vi "Dashboard Main.vi"() -> ()   [LabVIEW 2012]
uses:
  New_Framework_2013/AutoEnum.ctl
  <vilib>/event_ctls.llb/eventvkey.ctl
  <vilib>/Utility/config.llb/Read Key (String).vi
  <vilib>/Utility/config.llb/Read Key (I32).vi
  <vilib>/Utility/config.llb/Write Key (String).vi
  <vilib>/Utility/config.llb/Write Key (I32).vi
  <vilib>/Utility/config.llb/NI_LVConfig.lvlib
panel:
  out "Battery Value":dbl(slide) scale=0.0..14.0 scale format="%#_2e"
  out "Battery":sgl(graph)
  in  "Camera Settings":T1={"Frate Rate"=30, "Compression"=30, "Size"=1} {"Frate Rate" scale=1.0..30.0; "Size" items=["640x480", "320x240", "160x120"]}
  out "Mode":T2(ring)=enum."Auto Disabled"
  out "Camera IP":string
  out "Robot IP":string
  in  "Dashboard Tab":enum32{"Operation", "Test", "Checklist"}(tab)
  out "FrameworkVersion":string
  out "LauncherMotorValue":dbl
  out "Drive Loop Timing (ms)":u32
  out "ClimbState":string
  in  "AutoEnum":T3
  in  "Slider":dbl(slide) scale=0.0..100.0 scale format="%#_3g"
  in  "On/Off":bool caption="Solenoid"
  in  "Test Name":u16(ring) items=["Select the test to run...", "Example Test", "-------------------------------", "List of tests is built in robot code.", "Replace with your own automated tests."]
  in  "Test Tree":string(tree)
  in  "Motor":cluster{"Value":dbl, "Enable":bool} {"Value" scale=-1.0..1.0 scale format="%#_3g"}
  out "Progress":T4 {"Test Progress" scale=0.0..100.0}
  in  "Rev/Fwd":cluster{"Forward":bool, "Reverse":bool}
  in  "Ring":u16(ring) items=["Auto", "Fixed indoor", "Fixed outdoor 1", "Fixed outdoor 2", "Fixed fluorescent 1", "Fixed fluorescent 2", "Hold current"]
  in  "Listbox":i32(listbox)
  in  "Viewer":T5(tab)
  out "Mbps":dbl format="%#.1g"
  in  "Enable":bool
  in  "DB Camera Config":bool
  out "Mbps":bool
  out "fps":dbl format="%#.1g"
  out "Image Error Message":string="Timeout in Camera Communications"
  out "Camera Image":T6(plugin-control)
  out "Buttons 1":cluster{"1":bool, "2":bool, "3":bool}
  out "Kinect 1":cluster{"X":dbl, "Y":dbl, "Z":dbl} {"X" scale=1.0..-1.0; "Y" scale=1.0..-1.0; "Z" scale=1.0..-1.0}
  out "Buttons 2":cluster{"1":bool, "2":bool, "3":bool}
  out "Kinect 2":cluster{"X":dbl, "Y":dbl, "Z":dbl} {"X" scale=1.0..-1.0; "Y" scale=1.0..-1.0; "Z" scale=1.0..-1.0}
  out "Version":string
  out "Skeleton Picture":picture
  out "Players":i8
  out "Tree":string(tree)
  # "Drive & Motors"
  # "Robot IP:"
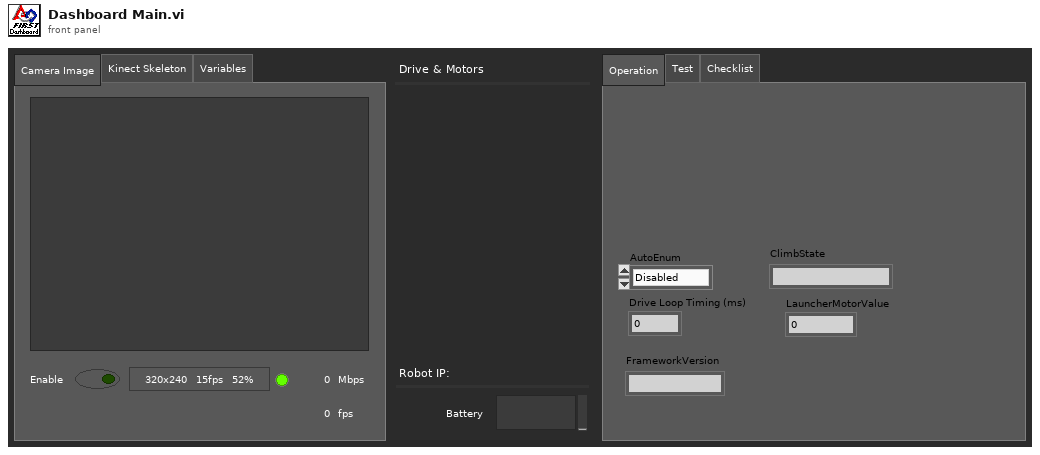
[diagram p1: front panel]
types:
  T1 = cluster{"Frate Rate":i32, "Compression":i32, "Size":u16}
  T2 = enum8{"Tele-Op Disabled", "Tele-Op Enabled", "Auto Disabled", "Auto Enabled", "Test Disabled", "Test Enabled", ""}
  T3 = typedef "AutoEnum.ctl" = enum16{"Disabled", "BackRight", "BackLeft", "CloseRight", "CloseLeft"}
  T4 = cluster{"Test Progress":u8, "Test Progress Text":string}
  T5 = enum32{"Camera Image", "Kinect Skeleton", "Variables"}
  T6 = typedef "IMAQ Image.ctl" = refnum<image>
  T7 = typedef "Image Type" = u32
  T8 = typedef "LVBoundsTypeDef.ctl" = cluster{"Width":u32, "Height":u32}
  T9 = typedef "SkeletonTrackState.ctl" = enum32{"NotTracked", "PositionOnly", "Tracked"}
  T10 = cluster{"TrackingState":u8[], "Position":cluster{"x":sgl, "y":sgl, "z":sgl}, cluster{"x":sgl, "y":sgl, "z":sgl, sgl}[], "TrackState":T9}
  T11 = cluster{cluster{"ScaledToPercentRange":dbl, "ScaledToPercentRange":dbl, "ScaledToPercentRange":dbl}, cluster{bool, bool, bool}}[]
  T12 = cluster{cluster{"ScaledToPercentRange":dbl, "ScaledToPercentRange":dbl, "ScaledToPercentRange":dbl}, cluster{bool, bool, bool}}
  T13 = cluster{"ScaledToPercentRange":dbl, "ScaledToPercentRange":dbl, "ScaledToPercentRange":dbl}
  T14 = typedef "LVRectTypeDef.ctl" = cluster{"Left":i16, "Top":i16, "Right":i16, "Bottom":i16}
  T15 = cluster{"Competition mode":bool, "Robot Link":bool, "Autonomous":bool, "Enabled":bool, "E-Stop":bool, "Simulated":bool, "TestMode":bool, "Docked Window":bool}
  T16 = typedef "NI_LVConfig.lvlib/Config Data RefNum.ctl" = refnum<k1>
  T17 = typedef "eventvkey.ctl" = enum16{"ASCII", "Enter", "Return", "Shift", "Ctrl", "Alt", "Cmd", "Opt", "Caps", "NumLock", "Clear", "Break", "Up", "Down", "Left", "Right", "Insert", "Delete", "Home", "End", "PageUp", "PageDown", "Escape", "Help", "Pause", "ScrollLock", "F1", "F2", "F3", "F4", "F5", "F6", "F7", "F8", "F9", "F10", "F11", "F12", "F13", "F14", "F15", "F16", "F17", "F18", "F19", "F20", "F21", "F22", "F23", "F24", "Play", "VolumeUp", "VolumeDown", "Mute", "Two Byte Char"}
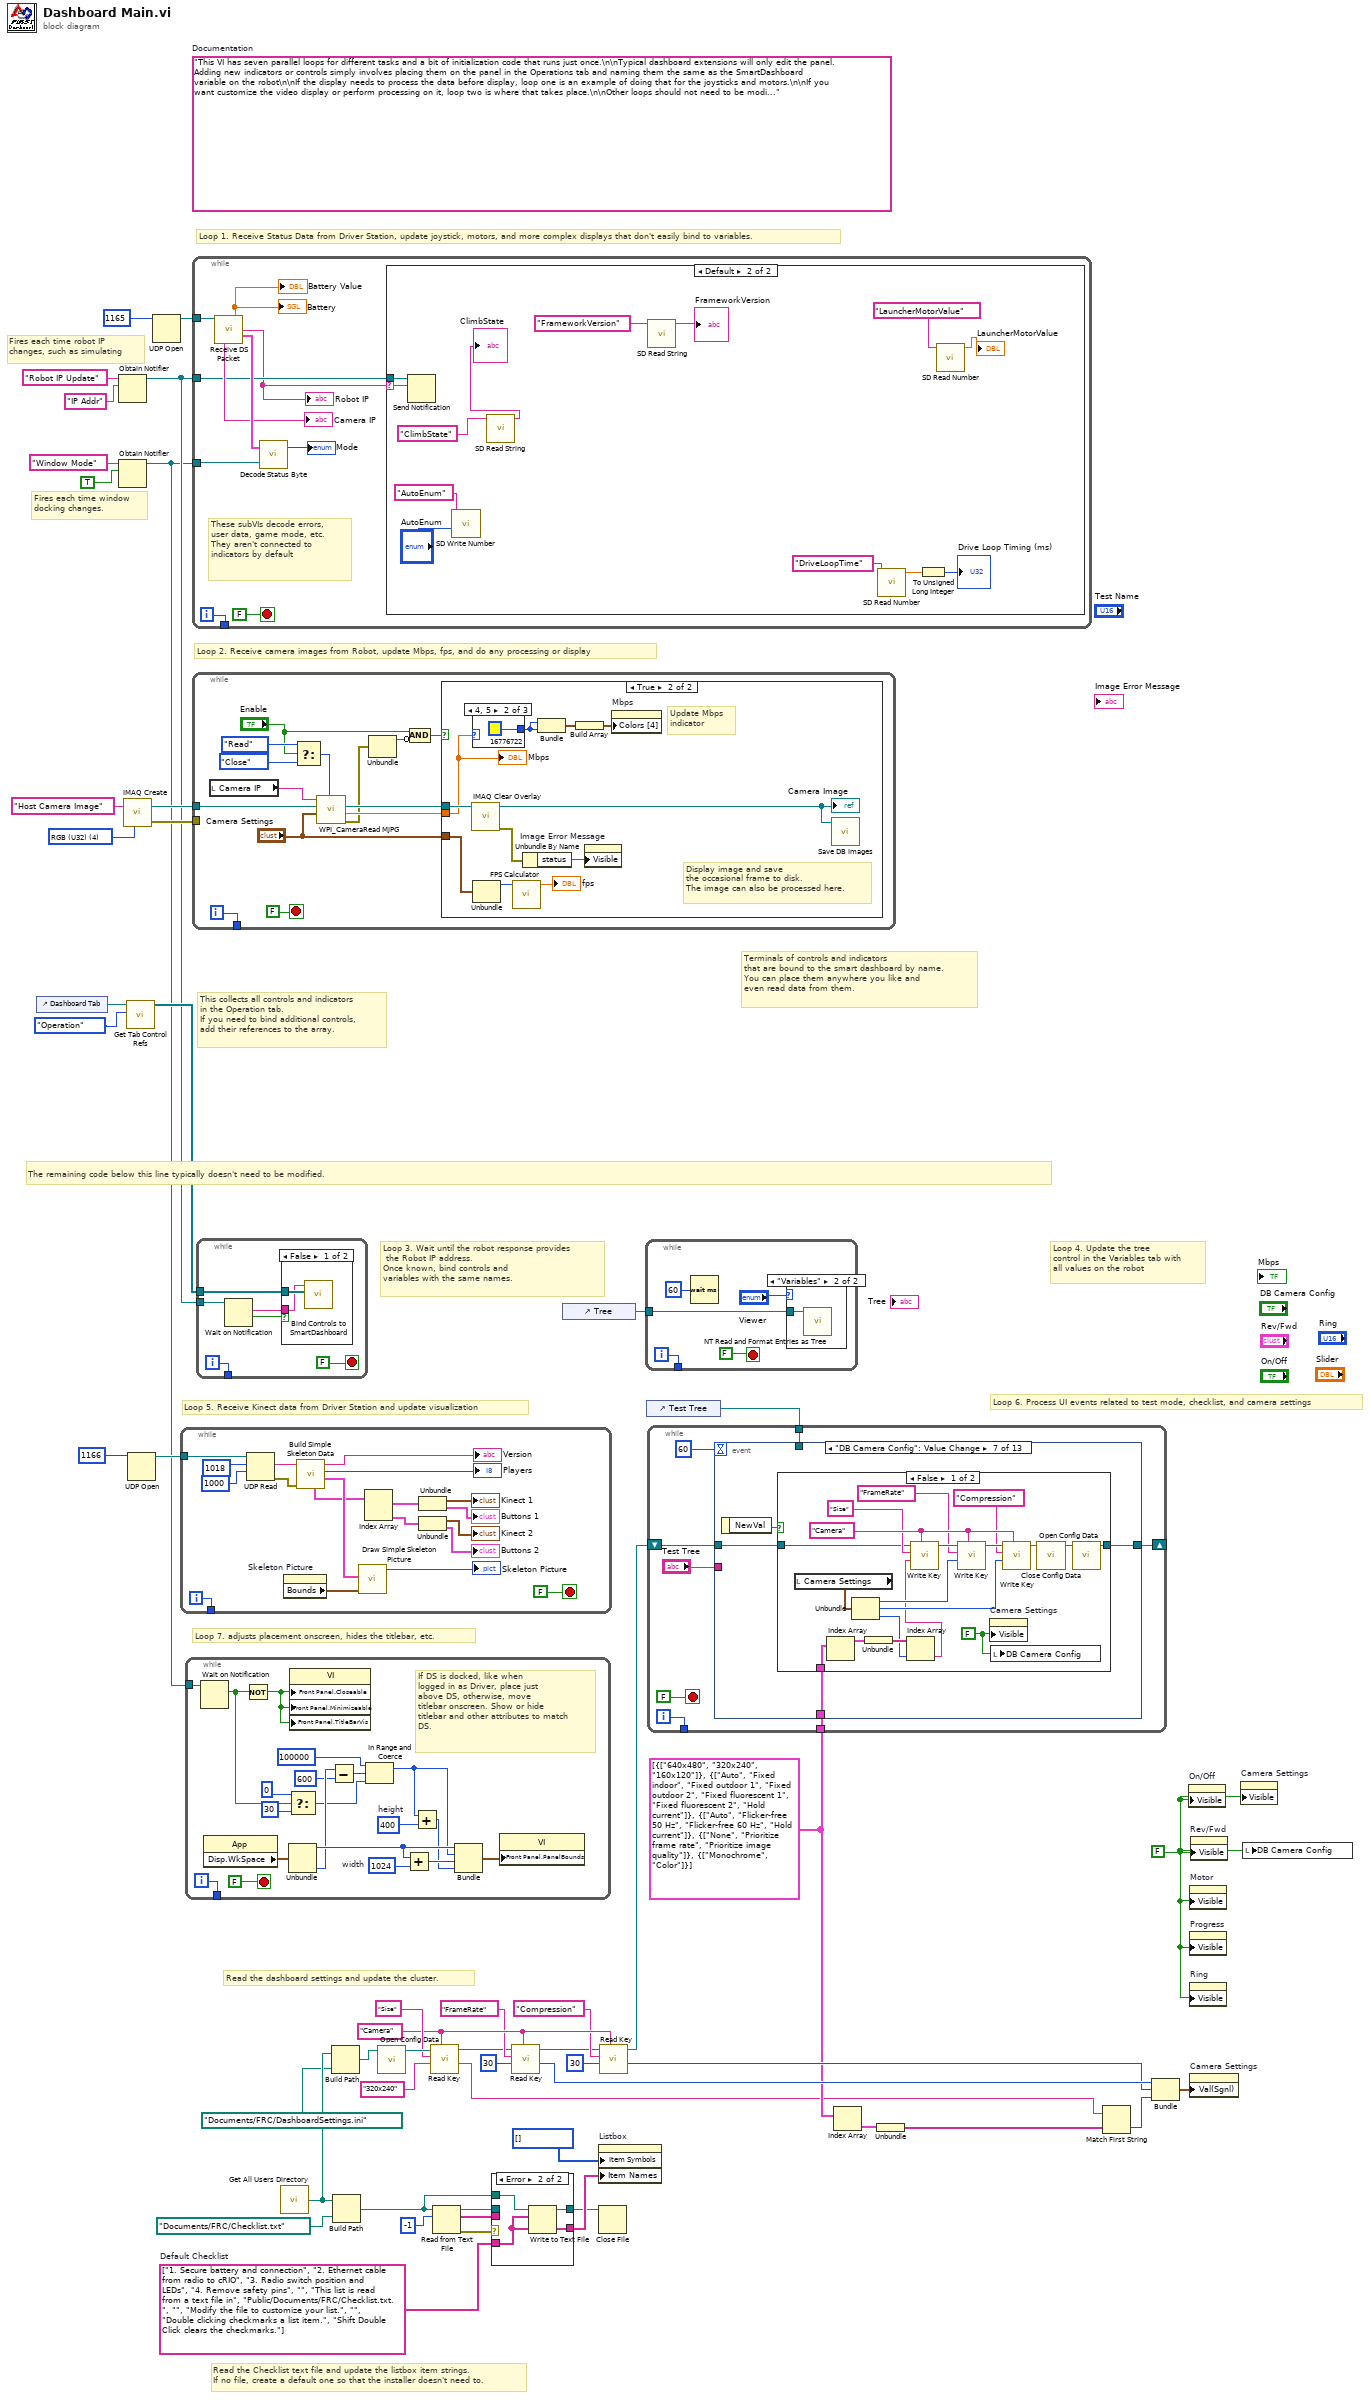
[diagram p0: block diagram]
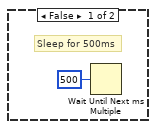
[diagram p3: hidden frame]
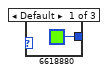
[diagram p4: hidden frame]
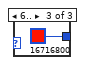
[diagram p5: hidden frame]
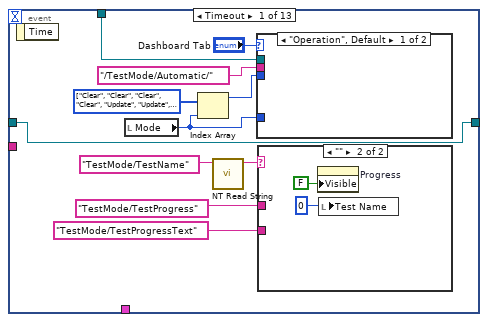
[diagram p7: hidden frame]
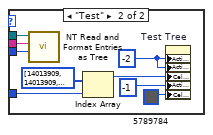
[diagram p8: hidden frame]
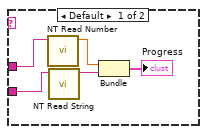
[diagram p9: hidden frame]
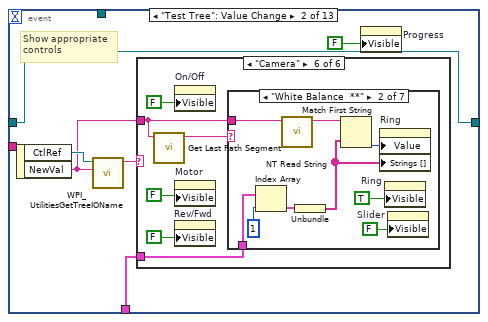
[diagram p10: hidden frame]
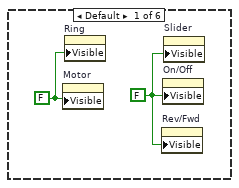
[diagram p11: hidden frame]
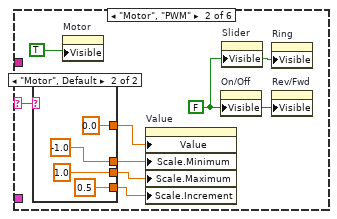
[diagram p12: hidden frame]
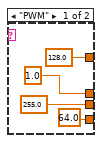
[diagram p13: hidden frame]
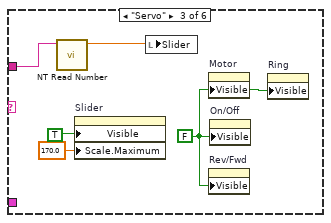
[diagram p14: hidden frame]
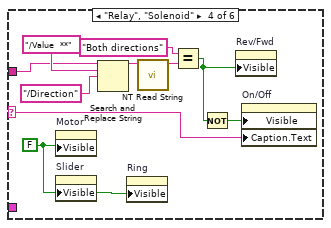
[diagram p15: hidden frame]
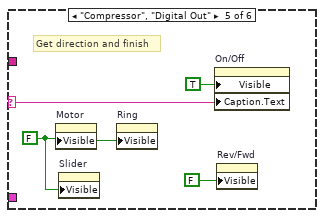
[diagram p16: hidden frame]
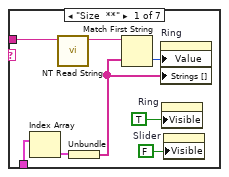
[diagram p17: hidden frame]
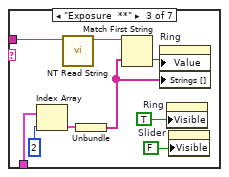
[diagram p18: hidden frame]
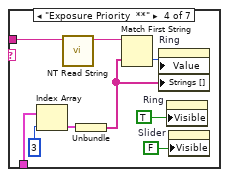
[diagram p19: hidden frame]
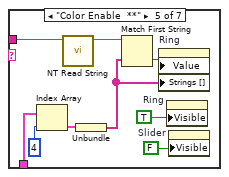
[diagram p20: hidden frame]
diagram:
  w21 = "Camera"
  w13 = cluster{string[]}[] [{["640x480", "320x240", "160x120"]}, {["Auto", "Fixed indoor", "Fixed outdoor 1", "Fixed outdoor 2", "Fixed fluorescent 1", "Fixed fluorescent 2", "Hold current"]}, {["Auto", "Flicker-free 50 Hz", "Flicker-free 60 Hz", "Hold current"]}, {["None", "Prioritize frame rate", "Prioritize image quality"]}, {["Monochrome", "Color"]}]
  w29 = string[] ["1. Secure battery and connection", "2. Ethernet cable from radio to cRIO", "3. Radio switch position and LEDs", "4. Remove safety pins", "", "This list is read from a text file in", "Public/Documents/FRC/Checklist.txt.", "", "Modify the file to customize your list.", "", "Double clicking checkmarks a list item.", "Shift Double Click clears the checkmarks."]  # Default Checklist
  w27 = FALSE ("Visible")
  (unwired) "This VI has seven parallel loops for different tasks and a bit of initialization code that runs just once.\n\nTypical dashboard extensions will only edit the panel. Adding new indicators or controls simply involves placing them on the panel in the Operations tab and naming them the same as the SmartDashboard variable on the robot\n\nIf the display needs to process the data before display, loop one is an example of doing that for the joysticks and motors.\n\nIf you want customize the video display or perform processing on it, loop two is where that takes place.\n\nOther loops should not need to be modified. They are pretty standard, and document the task they perform."  # Documentation
  w50 = T7 4 items=["Grayscale (U8)", "Grayscale (I16)", "Grayscale (SGL)", "Complex (CSG)", "RGB (U32)", "HSL (U32)", "RGB (U64)"] ("Image Type")
  # "Fires each time robot IP\nchanges, such as simulating"
  # "Fires each time window\ndocking changes."
  # "Read the Checklist text file and update the listbox item strings.\nIf no file, create a default one so that the installer doesn't need to."
  # "This collects all controls and indicators\nin the Operation tab.\nIf you need to bind additional controls,\nadd their references to the array."
  # "The remaining code below this line typically doesn't need to be modified."
  # "Loop 6. Process UI events related to test mode, checklist, and camera settings"
  # "Read the dashboard settings and update the cluster."
  # "Terminals of controls and indicators\nthat are bound to the smart dashboard by name.\nYou can place them anywhere you like and\neven read data from them."
  # "Loop 4. Update the tree\ncontrol in the Variables tab with\nall values on the robot"
  # "Loop 3. Wait until the robot response provides\n the Robot IP address.\nOnce known, bind controls and\nvariables with the same names."
  # "Loop 5. Receive Kinect data from Driver Station and update visualization"
  # "Loop 7. adjusts placement onscreen, hides the titlebar, etc."
  # "Loop 1. Receive Status Data from Driver Station, update joystick, motors, and more complex displays that don't easily bind to variables."
  # "Loop 2. Receive camera images from Robot, update Mbps, fps, and do any processing or display"
  n1 = control-ref of="Dashboard Tab"() -> (w43:refnum<vi>)
  n2 = Obtain Notifier(name (unnamed)="Robot IP Update", notification data type="IP Addr" ("name (unnamed)")) -> (notifier out=w40:refnum<notifier>)  [unwired: 2 in, 2 out]
  n3 = Obtain Notifier(name (unnamed)="Window Mode", notification data type=TRUE) -> (notifier out=w33:refnum<notifier>)  [unwired: 2 in, 2 out]
  n4 = call "IMAQ Create"("Image Name"="Host Camera Image", "Image Type"=w50) -> ("New Image"=w48:T6, "error out"=w47:errorcluster)  [unwired: 2 in, 1 out]
  n5 = call <vilib>:"Get Tab Control Refs.vi"("Page Index"=enum32{"Operation", "Test"}."Operation" ("Dashboard Tab"), "TabControl in"=w43) -> ("ControlsOnPage"=w44:refnum<vi>[])  [unwired: 9 in]
  n6 = UDP Open(11:u16 1166 ("port")) -> (port=w45:refnum<k16>)  [unwired: 2 in, 4 out]
  n7 = UDP Open(11:u16 1165 ("port")) -> (port=w51:refnum<k16>)  [unwired: 2 in, 4 out]
  n8 = while {
    tunnel: w45 -> [w69]
    tunnel: [w54] -> _
    i -> [w54]
    stop <- FALSE stop-if-true
    n9 = UDP Read(connection ID=w69, max size (548)=1018 ("bytes to read"), timeout ms (25000)=1000) -> (data out=w63:string, error out=w53:errorcluster)  [unwired: 1 in, 3 out]
    n10 = property on="Skeleton Picture" class="Pict"() -> ("Bounds"=w65:T8)  [unwired: 2 in, 2 out]
    n11 = call "Build Simple Skeleton Data.vi"("error in (no error)"=w53, "data in"=w63) -> ("Skeleton Data"=w64:T10, "NumPlayers"=→"Players":i8, "Version String"=→"Version":string, "Simple Joystick Info"=w61:T11)  [unwired: 5 in, 1 out]
    n12 = call "Draw Simple Skeleton Picture.vi"("Bounds"=w65, "Simple Skeleton"=w64) -> ("new picture out"=→"Skeleton Picture":picture)  [unwired: 9 in]
    n13 = Index Array(array=w61) -> (element #1=w60:T12, element #2=w59:T12)  [unwired: 2 in]
    n14 = Unbundle(w60) -> (→"Kinect 1":T13, →"Buttons 1":cluster{bool, bool, bool})
    n15 = Unbundle(w59) -> (→"Kinect 2":T13, →"Buttons 2":cluster{bool, bool, bool})
  }
  n16 = while {
    tunnel: w33 -> [w90]
    tunnel: [w88] -> _
    i -> [w88]
    stop <- FALSE stop-if-true
    w80 = 1024  # width
    w83 = 400  # height
    # "If DS is docked, like when\nlogged in as Driver, place just\nabove DS, otherwise, move\ntitlebar onscreen. Show or hide\ntitlebar and other attributes to match\nDS."
    n17 = Wait on Notification(notifier=w90) -> (notification=w75:bool)  [unwired: 3 in, 3 out]
    n18 = property class="App"() -> ("Disp.WkSpace"=w86:T14)  [unwired: 2 in, 2 out]
    n19 = Not(x=w75) -> (.not. x?=w89:bool)
    n20 = Unbundle(w86) -> ("Left"=w84:i16, "Bottom"=w81:i16)  [unwired: 2 out]
    n21 = Select(t=0, s=w75, f=30) -> (s? t:f=w74:i32)
    n22 = property class="VI"("Front Panel.Closeable"=w89, "Front Panel.Minimizeable"=w89, "Front Panel.TitleBarVis"=w89) -> ()  [unwired: 2 in, 2 out]
    n23 = Subtract(x=w81, y=600) -> (x-y=w78:i32)
    n24 = In Range and Coerce(upper limit=100000, x=w78, lower limit=w74) -> (coerced(x)=w72:i32)  [unwired: 1 out]
    n25 = Add(x=w84, y=w80) -> (x+y=w85:i32)
    n26 = Add(x=w72, y=w83) -> (x+y=w82:i32)
    n27 = Bundle("Left"=w84, w72, w85, w82) -> (w87:cluster{"Left":i16, i32, i32, i32})  [unwired: 1 out]
    n28 = property class="VI"("Front Panel.PanelBounds"=w87) -> ()  [unwired: 2 in, 2 out]
  }
  n29 = while {
    tunnel: w48 -> [w101]
    tunnel: w47 -> [_]
    tunnel: [w104] -> _
    i -> [w104]
    stop <- FALSE stop-if-true
    n30 = local read "Camera IP"() -> (w103:string)
    n31 = Select(t=enum16{"Read", "Reopen", "Close"}."Read" ("Operation"), s="Enable", f=enum16{"Read", "Reopen", "Close"}."Close" ("Operation")) -> (s? t:f=w96:enum16{"Read", "Reopen", "Close"})
    n32 = call <vilib>:"WPI_CameraRead MJPG.vi"("Operation"=w96, "Camera Settings"="Camera Settings", "Image"=w101, "address"=w103) -> ("error out"=w95:errorcluster, "Bandwidth (kbps)"=w99:dbl, "Image Out"=w100:T6)  [unwired: 5 in]
    n33 = Unbundle(w95) -> ("status"=w93:bool)  [unwired: 2 out]
    n34 = Compound Arithmetic op=AND("Enable", invert w93) -> (w92:bool)
    n35 = case shown="True" w92 {
      tunnel: "Camera Settings" -> [_ w108]
      tunnel: w100 -> [_ w111]
      tunnel: w99 -> [_ w110]
      frame False {
        # "Sleep for 500ms"
        n36 = Wait Until Next ms Multiple(millisecond multiple=u32 500) -> ()  [unwired: 1 out]
      }
      frame True {
        # "Display image and save\nthe occasional frame to disk.\nThe image can also be processed here."
        # "Update Mbps\nindicator"
        n37 = call "IMAQ Clear Overlay"("Image"=w111) -> ("error out"=w116:errorcluster, "Image Out"=w115:T6)  [unwired: 2 in, 7 out]
        "Camera Image" <- w115
        n38 = case shown="4, 5" w110 {
          tunnel: [u32 6618880 ("Color Box") u32 16776722 ("Color Box") u32 16716800 ("Color Box")] -> w112
          frame Default {
          }
          frame 4, 5 {
          }
          frame 6.. {
          }
        }
        n39 = Unbundle(w108) -> ("Frate Rate"=w107:i32)  [unwired: 2 out]
        n40 = call "FPS Calculator.vi"("Average Count"=w107) -> ("fps"=→"fps":dbl)  [unwired: 10 in]
        n41 = Unbundle By Name(w116) -> ("status"=w117:bool)
        n42 = Bundle("Color Box"=w112, "Color Box"=w112) -> (w114:cluster{"Color Box":u32, "Color Box":u32})  [unwired: 1 out]
        n43 = Build Array(w114) -> (w113:cluster{"Color Box":u32, "Color Box":u32}[])
        n44 = property on="Image Error Message" class="Str"("Visible"=w117) -> ()  [unwired: 2 in, 2 out]
        n45 = property on="Mbps" class="Bool (strict)"("Colors [4]"=w113) -> ()  [unwired: 2 in, 2 out]
        n46 = call "Save DB Images.vi"("Image"=w115) -> ()  [unwired: 2 in, 1 out]
        "Mbps" <- w110
      }
    }
  }
  n47 = while {
    tunnel: w51 -> [w128]
    tunnel: w40 -> [w122]
    tunnel: w33 -> [w126]
    tunnel: [w123] -> _
    i -> [w123]
    stop <- FALSE stop-if-true
    # "These subVIs decode errors, user data, game mode, etc.\nThey aren't connected to indicators by default"
    n48 = call "Receive DS Packet.vi"("Recv Socket"=w128) -> ("Battery"=→"Battery" →"Battery Value":sgl, "Robot IP Address"=w121:string, "Status"=w129:T15, "Camera IP Address"=→"Camera IP":string)  [unwired: 1 in, 10 out]
    "Robot IP" <- w121
    n49 = call "Decode Status Byte.vi"("Window Mode Notifier"=w126, "Status"=w129) -> ("Mode"=→"Mode":T2)  [unwired: 1 out]
    n50 = case shown="Default" w121 {
      selector: w121 -> [_ w142]
      tunnel: w122 -> [_ w143]
      frame "0.0.0.0" {
        # "Robot not responding, don't poll the variables"
      }
      frame Default {
        n51 = Send Notification(notification=w142, notifier=w143) -> ()  [unwired: 1 in, 2 out]
        n52 = call <vilib>:"SD Write Number.vi"("Numeric"="AutoEnum", "Name"="AutoEnum") -> ()  [unwired: 8 in, 2 out]
        n53 = call <vilib>:"SD Read String.vi"("Name"="ClimbState") -> ("String"=→"ClimbState":string)  [unwired: 8 in, 2 out]
        n54 = call <vilib>:"SD Read String.vi"("Name"="FrameworkVersion") -> ("String"=→"FrameworkVersion":string)  [unwired: 8 in, 2 out]
        n55 = call <vilib>:"SD Read Number.vi"("Name"="DriveLoopTime") -> ("Numeric"=w137:dbl)  [unwired: 8 in, 2 out]
        n56 = To Unsigned Long Integer(number=w137) -> (unsigned 32bit integer=→"Drive Loop Timing (ms)":u32)
        n57 = call <vilib>:"SD Read Number.vi"("Name"="LauncherMotorValue") -> ("Numeric"=→"LauncherMotorValue":dbl)  [unwired: 8 in, 2 out]
      }
    }
  }
  n58 = while {
    tunnel: w44 -> [w149]
    tunnel: w40 -> [w146]
    tunnel: [w144] -> _
    i -> [w144]
    stop <- FALSE stop-if-true
    n59 = Wait on Notification(notifier=w146) -> (notification=w145:string, timed out?=w147:bool)  [unwired: 3 in, 2 out]
    n60 = case shown="False" w147 {
      tunnel: w149 -> [w151 _]
      tunnel: w145 -> [w150 _]
      frame False {
        n61 = call <vilib>:"Bind Controls to SmartDashboard.vi"("Bound Control Refs"=w151, "Server IP Address"=w150) -> ()  [unwired: 10 in]
      }
      frame True {
      }
    }
  }
  n62 = call "Get All Users Directory.vi"() -> ("All User Path"=w26:path)
  n63 = Build Path(base path=w26, name or relative path=path "Documents/FRC/DashboardSettings.ini") -> (appended path=w25:path)
  n64 = Build Path(base path=w26, name or relative path=path "Documents/FRC/Checklist.txt") -> (appended path=w30:path)
  n65 = call <vilib>:"Open Config Data.vi"("configuration file path"=w25) -> ("refnum"=w24:T16)  [unwired: 8 in, 2 out]
  n66 = call-poly <vilib>:"Read Key.vi"("section"=w21, "default value"="320x240", "key"="Size", "refnum"=w24) -> ("value"=w11:string, "refnum out"=w6:T16)  [unwired: 2 in, 4 out]
  n67 = Read from Text File(file (use dialog)=w30, count=-1 ("timeout ms (25000)")) -> (refnum out=w8:refnum<file>, text=w31:string[], error out=w32:errorcluster)  [unwired: 2 in, 1 out]
  n68 = case shown="Error" w32 {
    tunnel: w31 -> [w153 _]
    tunnel: [w153 w155] -> w28
    tunnel: w29 -> [_ w155]
    tunnel: w30 -> [_ w156]
    tunnel: [w152 w154] -> w7
    tunnel: w8 -> [w152 _]
    frame No Error {
    }
    frame Error {
      n69 = Write to Text File(file (use dialog)=w156, text=w155) -> (refnum out=w154:refnum<file>)  [unwired: 2 in, 2 out]
    }
  }
  n70 = call-poly <vilib>:"Read Key.vi"("section"=w21, "default value"=30, "key"="FrameRate", "refnum"=w6) -> ("value"=w16:i32, "refnum out"=w5:T16)  [unwired: 1 in, 5 out]
  n71 = control-ref of="Tree"() -> (w2:refnum<vi>)
  n72 = property on="Listbox" class="LstBox (strict)"("Item Symbols"=i32[] [], "Item Names"=w28) -> ()  [unwired: 2 in, 2 out]
  n73 = Close File(refnum=w7) -> ()  [unwired: 1 in, 2 out]
  n74 = call-poly <vilib>:"Read Key.vi"("section"=w21, "default value"=30, "key"="Compression", "refnum"=w5) -> ("value"=w15:i32, "refnum out"=w3:T16)  [unwired: 1 in, 5 out]
  n75 = while {
    tunnel: [w158] -> _
    tunnel: w2 -> [w157]
    i -> [w158]
    stop <- FALSE stop-if-true
    n76 = Wait (ms)(milliseconds to wait=u32 60) -> ()  [unwired: 1 out]
    n77 = case shown="\"Variables\"" "Viewer" {
      tunnel: w157 -> [_ w162]
      frame Default {
      }
      frame "Variables" {
        n78 = call <vilib>:"NT Read and Format Entries as Tree.vi"("Tree Refnum"=w162) -> ()  [unwired: 9 in, 2 out]
      }
    }
  }
  n79 = control-ref of="Test Tree"() -> (w1:refnum<vi>)
  n80 = while {
    tunnel: w13 -> [w167]
    shift-right: [w166] -> _
    shift-left: w3 -> [w165]
    tunnel: [w164] -> _
    tunnel: w1 -> [w163]
    i -> [w164]
    stop <- FALSE stop-if-true
    n81 = event shown="[6] \"DB Camera Config\": Value Change" {
      selector: _ -> [_ _ _ _ _ _ _ _ _ _ _ _ _]
      dyn-events: _ -> [_ _ _ _ _ _ _ _ _ _ _ _ _]
      timeout: u32 60 ("milliseconds to wait") -> [_ _ _ _ _ _ _ _ _ _ _ _ _]
      tunnel: w163 -> [w177 _ _ _ _ _ _ _ _ _ _ _ _]
      tunnel: "Test Tree" -> [_ _ _ _ _ _ _ _ w371 w379 w381 w385 w393]
      tunnel: w167 -> [_ w199 _ _ _ _ w335 w365 _ _ _ _ _]
      tunnel: [w171 w198 _ w301 w309 w321 w334 w358 w370 w377 w380 w384 w392] -> w166
      tunnel: w165 -> [w171 w198 _ w301 w309 w321 w333 w358 w370 w377 w380 w384 w392]
      event Timeout {
        w176 = enum16{"Update", "Clear"}[] [enum."Clear", enum."Clear", enum."Clear", enum."Clear", enum."Update", enum."Update", enum."Clear"] items=["Update", "Clear"]
        n82 = event-data() -> ()  [unwired: 1 in, 1 out]
        n83 = local read "Mode"() -> (w174:T2)
        n84 = Index Array(array=w176, index=w174) -> (element=w175:enum16{"Update", "Clear"})
        n85 = call <vilib>:"NT Read String.vi"("Name"="TestMode/TestName") -> ("String"=w180:string)  [unwired: 9 in, 1 out]
        n86 = case shown="\"Operation\", Default" "Dashboard Tab" {
          tunnel: w177 -> [_ w190]
          tunnel: "/TestMode/Automatic/" ("Name Pattern") -> [_ w189]
          tunnel: w175 -> [_ w188]
          tunnel: w174 -> [_ w186]
          frame "Operation", Default {
          }
          frame "Test" {
            w185 = -2 ("Active Item:Row Number")
            n87 = call <vilib>:"NT Read and Format Entries as Tree.vi"("Operation"=w188, "Name Pattern"=w189, "Tree Refnum"=w190) -> ()  [unwired: 7 in, 2 out]
            n88 = Index Array(array=u32[] [14013909, 14013909, 14013909, 14013909, 14013909, 16777215, 14013909], index=w186) -> (element=w184:u32)
            n89 = property on="Test Tree" class="Tree (strict)"("Active Item Row Number"=w185, "ActiveColNum"=w185, "CellBG"=w184, "Active Item Row Number"=-1 ("Active Item:Row Number"), "CellBG"=u32 5789784 ("Color Box")) -> ()  [unwired: 2 in, 2 out]
          }
        }
        n90 = case shown="\"\"" w180 {
          tunnel: "TestMode/TestProgress" ("Name") -> [w192 _]
          tunnel: "TestMode/TestProgressText" ("Name") -> [w191 _]
          frame Default {
            n91 = call <vilib>:"NT Read Number.vi"("Name"=w192) -> ("Numeric"=w193:dbl)  [unwired: 9 in, 1 out]
            n92 = call <vilib>:"NT Read String.vi"("Name"=w191) -> ("String"=w194:string)  [unwired: 9 in, 1 out]
            n93 = Bundle("Numeric"=w193, "String"=w194) -> (→"Progress":cluster{"Numeric":dbl, "String":string})  [unwired: 1 in]
          }
          frame "" {
            n94 = property on="Progress" class="Clust (strict)"("Visible"=FALSE) -> ()  [unwired: 2 in, 2 out]
            n95 = local write "Test Name"(u16 0) -> ()
          }
        }
      }
      event "Test Tree": Value Change {
        # "Show appropriate\ncontrols"
        n96 = event-data() -> ("CtlRef"=w202:refnum<vi>, "NewVal"=w200:string)  [unwired: 1 in]
        n97 = call <vilib>:"WPI_UtilitiesGetTreeIOName.vi"("NewVal"=w200, "TreeControl in"=w202) -> ("I/O Name"=w203:string)  [unwired: 9 in]
        n98 = case shown="\"Camera\"" w203 {
          selector: w203 -> [_ w210 _ w228 w237 _]
          tunnel: w200 -> [_ _ w225 w227 _ w244]
          tunnel: w199 -> [_ _ _ _ _ w243]
          frame Default {
            w205 = FALSE ("Visible")
            w204 = FALSE ("Visible")
            n99 = property on="Motor" class="Clust (strict)"("Visible"=w204) -> ()  [unwired: 2 in, 2 out]
            n100 = property on="Ring" class="Ring (strict)"("Visible"=w204) -> ()  [unwired: 2 in, 2 out]
            n101 = property on="Rev/Fwd" class="Clust (strict)"("Visible"=w205) -> ()  [unwired: 2 in, 2 out]
            n102 = property on="On/Off" class="Bool (strict)"("Visible"=w205) -> ()  [unwired: 2 in, 2 out]
            n103 = property on="Slider" class="Slide (strict)"("Visible"=w205) -> ()  [unwired: 2 in, 2 out]
          }
          frame "Motor", "PWM" {
            w211 = FALSE ("Visible")
            n104 = case shown="\"Motor\", Default" w210 {
              tunnel: [1.0 ("Value") -1.0 ("Value")] -> w209
              tunnel: [255.0 ("Value") 1.0 ("Value")] -> w208
              tunnel: [128.0 ("Value") 0.0 ("Value")] -> w207
              tunnel: [64.0 ("Value") 0.5 ("Value")] -> w206
              frame "PWM" {
              }
              frame "Motor", Default {
              }
            }
            n105 = property on="Motor" class="Clust (strict)"("Visible"=TRUE) -> ()  [unwired: 2 in, 2 out]
            n106 = property on="Value" class="Slide (strict)"("Value"=w207, "Scale.Minimum"=w209, "Scale.Maximum"=w208, "Scale.Increment"=w206) -> ()  [unwired: 2 in, 2 out]
            n107 = property on="On/Off" class="Bool (strict)"("Visible"=w211) -> ()  [unwired: 2 in, 2 out]
            n108 = property on="Slider" class="Slide (strict)"("Visible"=w211) -> ()  [unwired: 2 in, 2 out]
            n109 = property on="Ring" class="Ring (strict)"("Visible"=w211) -> ()  [unwired: 2 in, 2 out]
            n110 = property on="Rev/Fwd" class="Clust (strict)"("Visible"=w211) -> ()  [unwired: 2 in, 2 out]
          }
          frame "Servo" {
            w223 = FALSE ("Visible")
            n111 = call <vilib>:"NT Read Number.vi"("Name"=w225) -> ("Numeric"=w224:dbl)  [unwired: 9 in, 1 out]
            n112 = property on="Slider" class="Slide (strict)"("Visible"=TRUE, "Scale.Maximum"=170.0 ("Scale.Range:Maximum")) -> ()  [unwired: 2 in, 2 out]
            n113 = local write "Slider"(w224) -> ()
            n114 = property on="Motor" class="Clust (strict)"("Visible"=w223) -> ()  [unwired: 2 in, 2 out]
            n115 = property on="Rev/Fwd" class="Clust (strict)"("Visible"=w223) -> ()  [unwired: 2 in, 2 out]
            n116 = property on="On/Off" class="Bool (strict)"("Visible"=w223) -> ()  [unwired: 2 in, 2 out]
            n117 = property on="Ring" class="Ring (strict)"("Visible"=w223) -> ()  [unwired: 2 in, 2 out]
          }
          frame "Relay", "Solenoid" {
            w226 = FALSE ("Visible")
            n118 = property on="Motor" class="Clust (strict)"("Visible"=w226) -> ()  [unwired: 2 in, 2 out]
            n119 = property on="Slider" class="Slide (strict)"("Visible"=w226) -> ()  [unwired: 2 in, 2 out]
            n120 = Search and Replace String(input string=w227, search string="/Value  **", replace string="/Direction") -> (result string=w233:string)  [unwired: 5 in, 3 out]
            n121 = property on="Ring" class="Ring (strict)"("Visible"=w226) -> ()  [unwired: 2 in, 2 out]
            n122 = call <vilib>:"NT Read String.vi"("Name"=w233) -> ("String"=w231:string)  [unwired: 9 in, 1 out]
            n123 = Equal?(x="Both directions", y=w231) -> (x = y?=w229:bool)
            n124 = Not(x=w229) -> (.not. x?=w230:bool)
            n125 = property on="Rev/Fwd" class="Clust (strict)"("Visible"=w229) -> ()  [unwired: 2 in, 2 out]
            n126 = property on="On/Off" class="Bool (strict)"("Visible"=w230, "Caption.Text"=w228) -> ()  [unwired: 2 in, 2 out]
          }
          frame "Compressor", "Digital Out" {
            w236 = FALSE ("Visible")
            # "Get direction and finish"
            n127 = property on="Motor" class="Clust (strict)"("Visible"=w236) -> ()  [unwired: 2 in, 2 out]
            n128 = property on="Slider" class="Slide (strict)"("Visible"=w236) -> ()  [unwired: 2 in, 2 out]
            n129 = property on="Ring" class="Ring (strict)"("Visible"=w236) -> ()  [unwired: 2 in, 2 out]
            n130 = property on="On/Off" class="Bool (strict)"("Visible"=TRUE, "Caption.Text"=w237) -> ()  [unwired: 2 in, 2 out]
            n131 = property on="Rev/Fwd" class="Clust (strict)"("Visible"=FALSE) -> ()  [unwired: 2 in, 2 out]
          }
          frame "Camera" {
            n132 = call <vilib>:"Get Last Path Segment.vi"("String in"=w244) -> ("String out"=w245:string)  [unwired: 10 in]
            n133 = property on="On/Off" class="Bool (strict)"("Visible"=FALSE) -> ()  [unwired: 2 in, 2 out]
            n134 = property on="Motor" class="Clust (strict)"("Visible"=FALSE) -> ()  [unwired: 2 in, 2 out]
            n135 = property on="Rev/Fwd" class="Clust (strict)"("Visible"=FALSE) -> ()  [unwired: 2 in, 2 out]
            n136 = case shown="\"White Balance  **\"" w245 {
              tunnel: w244 -> [w251 w260 w269 w278 w287 _ w293]
              tunnel: w243 -> [w249 w257 w266 w275 w284 _ _]
              frame "Size  **" {
                n137 = Index Array(array=w249) -> (element=w248:cluster{string[]})  [unwired: 1 in]
                n138 = call <vilib>:"NT Read String.vi"("Name"=w251) -> ("String"=w250:string)  [unwired: 9 in, 1 out]
                n139 = Unbundle(w248) -> (w246:string[])
                n140 = Match First String(2:w246, 3:w250) -> (0:w247:i32)  [unwired: 1 out]
                n141 = property on="Ring" class="Ring (strict)"("Value"=w247, "Strings []"=w246) -> ()  [unwired: 2 in, 2 out]
                n142 = property on="Ring" class="Ring (strict)"("Visible"=TRUE) -> ()  [unwired: 2 in, 2 out]
                n143 = property on="Slider" class="Slide (strict)"("Visible"=FALSE) -> ()  [unwired: 2 in, 2 out]
              }
              frame "White Balance  **" {
                n144 = Index Array(array=w257, index=1) -> (element=w258:cluster{string[]})
                n145 = call <vilib>:"NT Read String.vi"("Name"=w260) -> ("String"=w259:string)  [unwired: 9 in, 1 out]
                n146 = Unbundle(w258) -> (w255:string[])
                n147 = Match First String(2:w255, 3:w259) -> (0:w254:i32)  [unwired: 1 out]
                n148 = property on="Ring" class="Ring (strict)"("Value"=w254, "Strings []"=w255) -> ()  [unwired: 2 in, 2 out]
                n149 = property on="Ring" class="Ring (strict)"("Visible"=TRUE) -> ()  [unwired: 2 in, 2 out]
                n150 = property on="Slider" class="Slide (strict)"("Visible"=FALSE) -> ()  [unwired: 2 in, 2 out]
              }
              frame "Exposure  **" {
                n151 = Index Array(array=w266, index=2) -> (element=w267:cluster{string[]})
                n152 = call <vilib>:"NT Read String.vi"("Name"=w269) -> ("String"=w268:string)  [unwired: 9 in, 1 out]
                n153 = Unbundle(w267) -> (w263:string[])
                n154 = Match First String(2:w263, 3:w268) -> (0:w264:i32)  [unwired: 1 out]
                n155 = property on="Ring" class="Ring (strict)"("Value"=w264, "Strings []"=w263) -> ()  [unwired: 2 in, 2 out]
                n156 = property on="Ring" class="Ring (strict)"("Visible"=TRUE) -> ()  [unwired: 2 in, 2 out]
                n157 = property on="Slider" class="Slide (strict)"("Visible"=FALSE) -> ()  [unwired: 2 in, 2 out]
              }
              frame "Exposure Priority  **" {
                n158 = Index Array(array=w275, index=3) -> (element=w276:cluster{string[]})
                n159 = call <vilib>:"NT Read String.vi"("Name"=w278) -> ("String"=w277:string)  [unwired: 9 in, 1 out]
                n160 = Unbundle(w276) -> (w272:string[])
                n161 = Match First String(2:w272, 3:w277) -> (0:w273:i32)  [unwired: 1 out]
                n162 = property on="Ring" class="Ring (strict)"("Value"=w273, "Strings []"=w272) -> ()  [unwired: 2 in, 2 out]
                n163 = property on="Ring" class="Ring (strict)"("Visible"=TRUE) -> ()  [unwired: 2 in, 2 out]
                n164 = property on="Slider" class="Slide (strict)"("Visible"=FALSE) -> ()  [unwired: 2 in, 2 out]
              }
              frame "Color Enable  **" {
                n165 = Index Array(array=w284, index=4) -> (element=w285:cluster{string[]})
                n166 = call <vilib>:"NT Read String.vi"("Name"=w287) -> ("String"=w286:string)  [unwired: 9 in, 1 out]
                n167 = Unbundle(w285) -> (w281:string[])
                n168 = Match First String(2:w281, 3:w286) -> (0:w282:i32)  [unwired: 1 out]
                n169 = property on="Ring" class="Ring (strict)"("Value"=w282, "Strings []"=w281) -> ()  [unwired: 2 in, 2 out]
                n170 = property on="Ring" class="Ring (strict)"("Visible"=TRUE) -> ()  [unwired: 2 in, 2 out]
                n171 = property on="Slider" class="Slide (strict)"("Visible"=FALSE) -> ()  [unwired: 2 in, 2 out]
              }
              frame Default {
                n172 = property on="Ring" class="Ring (strict)"("Visible"=FALSE) -> ()  [unwired: 2 in, 2 out]
                n173 = property on="Slider" class="Slide (strict)"("Visible"=FALSE) -> ()  [unwired: 2 in, 2 out]
              }
              frame "Brightness  **", "Color Level  **", "Compression  **", "FPS  **", "Sharpness  **" {
                n174 = call <vilib>:"NT Read Number.vi"("Name"=w293) -> ("Numeric"=w292:dbl)  [unwired: 9 in, 1 out]
                n175 = local write "Slider"(w292) -> ()
                n176 = property on="Slider" class="Slide (strict)"("Visible"=TRUE, "Scale.Maximum"=100.0 ("Scale.Range:Maximum")) -> ()  [unwired: 2 in, 2 out]
                n177 = property on="Ring" class="Ring (strict)"("Visible"=FALSE) -> ()  [unwired: 2 in, 2 out]
              }
            }
          }
        }
        n178 = property on="Progress" class="Clust (strict)"("Visible"=FALSE) -> ()  [unwired: 2 in, 2 out]
      }
      event "Test Name": Mouse Enter {
        # "Populate the ring with the list of tests"
        n179 = event-data() -> ()  [unwired: 1 in, 1 out]
        n180 = call <vilib>:"NT Read String Array.vi"("Name"="TestMode/TestList") -> ("String Array"=w300:string[])  [unwired: 9 in, 1 out]
        n181 = Build Array (concatenate)("Select the test to run...", w300) -> (w299:string[])
        n182 = property on="Test Name" class="Ring (strict)"("Strings []"=w299) -> ()  [unwired: 2 in, 2 out]
      }
      event "Test Name": Value Change {
        w302 = FALSE ("Visible")
        # "Tell the robot the test name to run"
        n183 = event-data() -> ("NewVal"=w306:u16)  [unwired: 1 in]
        n184 = property on="Test Name" class="Ring (strict)"() -> ("Strings []"=w307:string[])  [unwired: 2 in, 2 out]
        n185 = local write "Progress"(T4 {"Test Progress"=0, "Test Progress Text"=""} ("Progress")) -> ()
        n186 = Index Array(array=w307, index=w306) -> (element=w305:string)
        n187 = call <vilib>:"NT Write String.vi"("String"=w305, "Name"="TestMode/TestName") -> ()  [unwired: 9 in, 1 out]
        n188 = property on="Progress" class="Clust (strict)"("Visible"=TRUE) -> ()  [unwired: 2 in, 2 out]
        n189 = property on="Motor" class="Clust (strict)"("Visible"=w302) -> ()  [unwired: 2 in, 2 out]
        n190 = property on="Slider" class="Slide (strict)"("Visible"=w302) -> ()  [unwired: 2 in, 2 out]
        n191 = property on="On/Off" class="Bool (strict)"("Visible"=w302) -> ()  [unwired: 2 in, 2 out]
        n192 = property on="Rev/Fwd" class="Clust (strict)"("Visible"=w302) -> ()  [unwired: 2 in, 2 out]
        n193 = property on="Ring" class="Ring (strict)"("Visible"=w302) -> ()  [unwired: 2 in, 2 out]
      }
      event "Listbox": Double Click {
        n194 = event-data() -> ("PlatMods.Shift"=w310:bool, "Row"=w312:i32)  [unwired: 1 in]
        n195 = case shown="False" w310 {
          tunnel: w312 -> [w316 _]
          tunnel: 1 -> [w315 _]
          frame False {
            n196 = property on="Listbox" class="LstBox (strict)"() -> ("Item Symbols"=w314:i32[])  [unwired: 2 in, 2 out]
            n197 = Replace Array Subset(array=w314, new element=w315, index=w316) -> (w313:i32[])
            n198 = property on="Listbox" class="LstBox (strict)"("Item Symbols"=w313) -> ()  [unwired: 2 in, 2 out]
          }
          frame True {
            w317 = 0 ("Top Row")
            n199 = property on="Listbox" class="LstBox (strict)"() -> ("Number of Rows"=w319:u32)  [unwired: 2 in, 2 out]
            n200 = Initialize Array(0, w319) -> (w318:i32[])
            n201 = property on="Listbox" class="LstBox (strict)"("Top Row"=w317, "Value"=w317, "Item Symbols"=w318) -> ()  [unwired: 2 in, 2 out]
          }
        }
      }
      event "Listbox": Key Down {
        n202 = event-data() -> ("VKey"=w323:T17)  [unwired: 1 in]
        n203 = case shown="\"Left\", \"Right\"" w323 {
          selector: w323 -> [w328 _]
          tunnel: eventvkey."Left" ("VKey") -> [w326 _]
          frame "Left", "Right" {
            n204 = Equal?(x=w326, y=w328) -> (x = y?=w327:bool)
            n205 = Select(t=0, s=w327, f=1) -> (s? t:f=w329:i32)
            n206 = property on="Listbox" class="LstBox (strict)"() -> ("Item Symbols"=w332:i32[])  [unwired: 2 in, 2 out]
            n207 = Replace Array Subset(array=w332, new element=w329, index="Listbox") -> (w331:i32[])
            n208 = property on="Listbox" class="LstBox (strict)"("Item Symbols"=w331) -> ()  [unwired: 2 in, 2 out]
          }
          frame Default {
          }
        }
      }
      event "DB Camera Config": Value Change {
        n209 = event-data() -> ("NewVal"=w336:bool)  [unwired: 1 in]
        n210 = case shown="False" w336 {
          tunnel: w335 -> [w345 _]
          tunnel: [w338 w356] -> w334
          tunnel: w333 -> [w337 w356]
          frame False {
            w352 = "Camera"
            w355 = FALSE ("Visible")
            n211 = local read "Camera Settings"() -> (w344:T1)
            n212 = Index Array(array=w345) -> (element=w348:cluster{string[]})  [unwired: 1 in]
            n213 = Unbundle(w344) -> ("Frate Rate"=w343:i32, "Compression"=w342:i32, "Size"=w346:u16)
            n214 = Unbundle(w348) -> (w347:string[])
            n215 = Index Array(array=w347, index=w346) -> (element=w341:string)
            n216 = call-poly <vilib>:"Write Key.vi"("section"=w352, "value"=w341, "key"="Size", "refnum"=w337) -> ("refnum out"=w354:T16)  [unwired: 2 in, 5 out]
            n217 = call-poly <vilib>:"Write Key.vi"("section"=w352, "value"=w343, "key"="FrameRate", "refnum"=w354) -> ("refnum out"=w353:T16)  [unwired: 1 in, 6 out]
            n218 = property on="Camera Settings" class="Clust (strict)"("Visible"=w355) -> ()  [unwired: 2 in, 2 out]
            n219 = local write "DB Camera Config"(w355) -> ()
            n220 = call-poly <vilib>:"Write Key.vi"("section"=w352, "value"=w342, "key"="Compression", "refnum"=w353) -> ("refnum out"=w339:T16)  [unwired: 1 in, 6 out]
            n221 = call <vilib>:"Close Config Data.vi"("refnum"=w339) -> ("file path"=w340:path)  [unwired: 2 in, 8 out]
            n222 = call <vilib>:"Open Config Data.vi"("configuration file path"=w340) -> ("refnum"=w338:T16)  [unwired: 8 in, 2 out]
          }
          frame True {
            n223 = property on="Camera Settings" class="Clust (strict)"("Visible"=TRUE) -> ()  [unwired: 2 in, 2 out]
          }
        }
      }
      event "Camera Settings": Value Change {
        n224 = event-data() -> ("NewVal"=w369:T1)  [unwired: 1 in]
        n225 = Index Array(array=w365) -> (element=w364:cluster{string[]})  [unwired: 1 in]
        n226 = Unbundle(w369) -> ("Frate Rate"=w360:i32, "Compression"=w359:i32, "Size"=w362:u16)
        n227 = Unbundle(w364) -> (w363:string[])
        n228 = Index Array(array=w363, index=w362) -> (element=w361:string)
        n229 = Format Into String(format string="%s   %dfps   %d%%", w361, w360, w359) -> (resulting string=w366:string)  [unwired: 2 in, 1 out]
        n230 = Build Array(w366) -> (w367:string[])
        n231 = property on="DB Camera Config" class="Bool (strict)"("Strings [4]"=w367) -> ()  [unwired: 2 in, 2 out]
      }
      event "Motor.Enable": Value Change {
        n232 = event-data() -> ("NewVal"=w375:bool)  [unwired: 1 in]
        n233 = Unbundle("Motor") -> ("Value"=w374:dbl)  [unwired: 1 out]
        n234 = Select(t=w374, s=w375, f=0.0) -> (s? t:f=w372:dbl)
        n235 = call <vilib>:"NT Write Number.vi"("Numeric"=w372, "Name"=w371) -> ()  [unwired: 9 in, 1 out]
      }
      event "Slider": Value Change {
        n236 = event-data() -> ("NewVal"=w378:dbl)  [unwired: 1 in]
        n237 = call <vilib>:"NT Write Number.vi"("Numeric"=w378, "Name"=w379) -> ()  [unwired: 9 in, 1 out]
      }
      event "On/Off": Value Change {
        n238 = event-data() -> ("NewVal"=w383:bool)  [unwired: 1 in]
        n239 = Boolean To (0,1)(Boolean=w383) -> (0, 1=w382:i16)
        n240 = call <vilib>:"NT Write Number.vi"("Numeric"=w382, "Name"=w381) -> ()  [unwired: 9 in, 1 out]
      }
      event "Rev/Fwd": Value Change {
        n241 = event-data() -> ("NewVal.Forward"=w391:bool, "NewVal.Reverse"=w390:bool)  [unwired: 1 in]
        n242 = Boolean To (0,1)(Boolean=w391) -> (0, 1=w387:i16)
        n243 = Boolean To (0,1)(Boolean=w390) -> (0, 1=w389:i16)
        n244 = Negate(x=w389) -> (-x=w388:i16)
        n245 = Add(x=w387, y=w388) -> (x+y=w386:i16)
        n246 = call <vilib>:"NT Write Number.vi"("Numeric"=w386, "Name"=w385) -> ()  [unwired: 9 in, 1 out]
      }
      event "Ring": Value Change {
        n247 = event-data() -> ("NewVal"=w395:u16)  [unwired: 1 in]
        n248 = property on="Ring" class="Ring (strict)"() -> ("Strings []"=w396:string[])  [unwired: 2 in, 2 out]
        n249 = Index Array(array=w396, index=w395) -> (element=w394:string)
        n250 = call <vilib>:"NT Write String.vi"("String"=w394, "Name"=w393) -> ()  [unwired: 9 in, 1 out]
      }
    }
  }
  n251 = Index Array(array=w13) -> (element=w14:cluster{string[]})  [unwired: 1 in]
  n252 = Unbundle(w14) -> (w12:string[])
  n253 = Match First String(2:w12, 3:w11) -> (0:w10:i32)  [unwired: 1 out]
  n254 = Bundle("value"=w16, "value"=w15, "index"=w10) -> (w4:cluster{"value":i32, "value":i32, "index":i32})  [unwired: 1 out]
  n255 = property on="On/Off" class="Bool (strict)"("Visible"=w27) -> ()  [unwired: 2 in, 2 out]
  n256 = property on="Motor" class="Clust (strict)"("Visible"=w27) -> ()  [unwired: 2 in, 2 out]
  n257 = property on="Progress" class="Clust (strict)"("Visible"=w27) -> ()  [unwired: 2 in, 2 out]
  n258 = property on="Ring" class="Ring (strict)"("Visible"=w27) -> ()  [unwired: 2 in, 2 out]
  n259 = property on="Camera Settings" class="Clust (strict)"("Val(Sgnl)"=w4) -> ()  [unwired: 2 in, 2 out]
  n260 = property on="Rev/Fwd" class="Clust (strict)"("Visible"=w27) -> ()  [unwired: 2 in, 2 out]
  n261 = property on="Camera Settings" class="Clust (strict)"("Visible"=w27) -> ()  [unwired: 2 in, 2 out]
  n262 = local write "DB Camera Config"(w27) -> ()
